vi "Main.vi"(0 "Page Selector":T1, 1 "Code":i32 min=0 max=40000, 4 "Work Area":T2(tab), 5 "Mode Selector":T3, 7 "Instrument Setting":T4={"Error Percentage"=20.0} {"Error Percentage" min=0.0 max=100.0}, 9 "INL Method":T5, 11 "Error In":errorcluster, 12 "Input Voltage Parameters":T6={"Voltage Max"=5.0, "Voltage Min"=0.0, "No.of bits"=3.0} {"No.of bits" min=1.0}) -> (3 "DNL Value":dbl, 6 "DNL Graph":dbl[](graph), 8 "INL Graph":dbl[](graph), 10 "Ideal Transfer Function":cluster{"Analog Voltage":dbl[], dbl[]}(graph), 13 "INL Value":dbl, 14 "Status":string, 15 "Error Out":errorcluster)   [LabVIEW 2023]
doc: "This VI serves as the main entry point for the software framework used to measure INL and DNL for ADC and DAC devices. It initializes the GUI, loads necessary resources, handles user interactions to perform and display measurements."
uses:
  Typedef/INL Method.ctl
  Typedef/Page Selector.ctl
  Typedef/Mode Selector.ctl
  Typedef/Input Voltage Parameters.ctl
  Typedef/Instrument Setting.ctl
  Typedef/Queue Operation.ctl
  Typedef/INL and DNL calculation data.ctl
  Classes/Application/Application.lvclass
  Typedef/Class Details.ctl
  Typedef/Transfer Function.ctl
  Typedef/User Event Operations.ctl
panel:
  in  "Input":bool
  in  "Back":bool
  out "Device Result":string
  # "INL AND DNL TESTS FOR DAC AND ADCs"
  # "Purpose\nThis tool measures Integral Non-Linearity (INL) and Differential Non-Linearity (DNL) of ADCs and DACs, ensuring accurate linearity performance for various applications.\n\nINL and DNL Definitions\nINL (Integral Non-Linearity): Deviation of the converter's actual transfer function from an ideal straight line.\nDNL (Differential Non-Linearity): Deviation between adjacent digital output levels, indicating the uniformity of steps.\n\nA DNL of greater than -1 LSB will guarantee monotonicity and no missing codes.\nMonotonicity\nA device is termed monotonic if the analog output always increases or remains constant as the digital input increases. If the DNL is less than -1 LSB, the transfer function is non-monotonic."
  # "Fig: DNL calculation for ADC"
  # "Please select the mode of the device"
  # "Note: Instrument currently does not work for DAC devices"
  # "Choose the type of INL Measurement"
  # "Specify the error percentage in the limit 0 - 100%"
  # "Please enter the input voltage parameters to generate ideal transfer function"
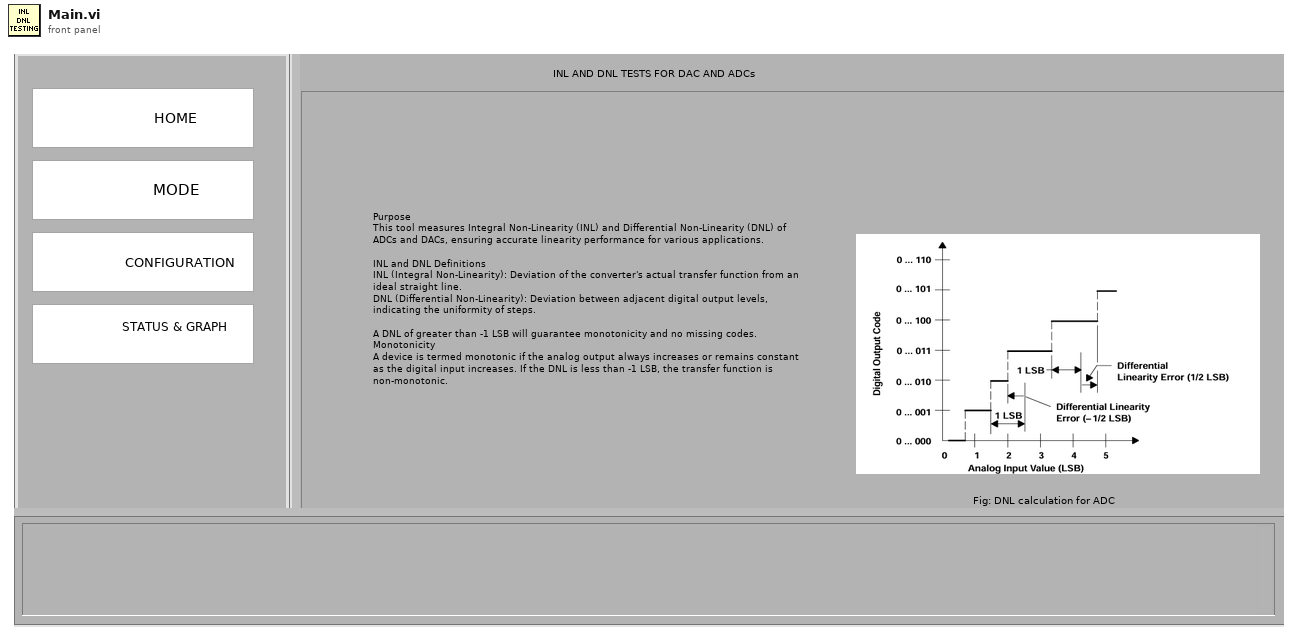
[diagram p1: front panel]
types:
  T1 = typedef "Page Selector.ctl" = cluster{"Mode":bool, "Configuration":bool, "Result":bool, "Home":bool}
  T2 = enum32{"Home Page", "Mode Page", "Configuration Page", "Input Page", "Result Page"}
  T3 = typedef "Mode Selector.ctl" = cluster{"DAC":bool, "ADC":bool}
  T4 = typedef "Instrument Setting.ctl" = cluster{"Error Percentage":dbl}
  T5 = typedef "INL Method.ctl" = enum16{"Best Fit", "End Point"}
  T6 = typedef "Input Voltage Parameters.ctl" = cluster{"Voltage Max":dbl, "Voltage Min":dbl, "No.of bits":dbl}
  T7 = typedef "User Event Operations.ctl" = enum16{"Initialize", "Read", "Write"}
  T8 = typedef "INL and DNL calculation data.ctl" = cluster{"Input Values":T6, "DNL":dbl, "INL":dbl, "DNL Graph":dbl[], "Code":i32, "INL Graph":dbl[], "Error Percentage":dbl, "Status History":string[], "Status Limit":i32, "Statusbar":string, "Active Class":refnum<class "Application.lvclass">, "INL Method":T5, "List of Classes":T9[], "Selected Mode":string, "Base Class":refnum<class "Application.lvclass">, "Transform Function":T10, "Monotonic?":bool, "Device Result":string}
  T9 = typedef "Class Details.ctl" = cluster{"Class Name":string, "Class Data":refnum<class "Application.lvclass">}
  T10 = typedef "Transfer Function.ctl" = cluster{"Ideal voltage":dbl[], "Digital Code":dbl[]}
  T11 = typedef "Queue Operation.ctl" = enum16{"Create & Enqueue N", "Enqueue N", "Dequeue", "Enstack N", "Flush", "Release"}
  T12 = typedef "Queue Element.ctl" = cluster{"State":string, "Data":variant}
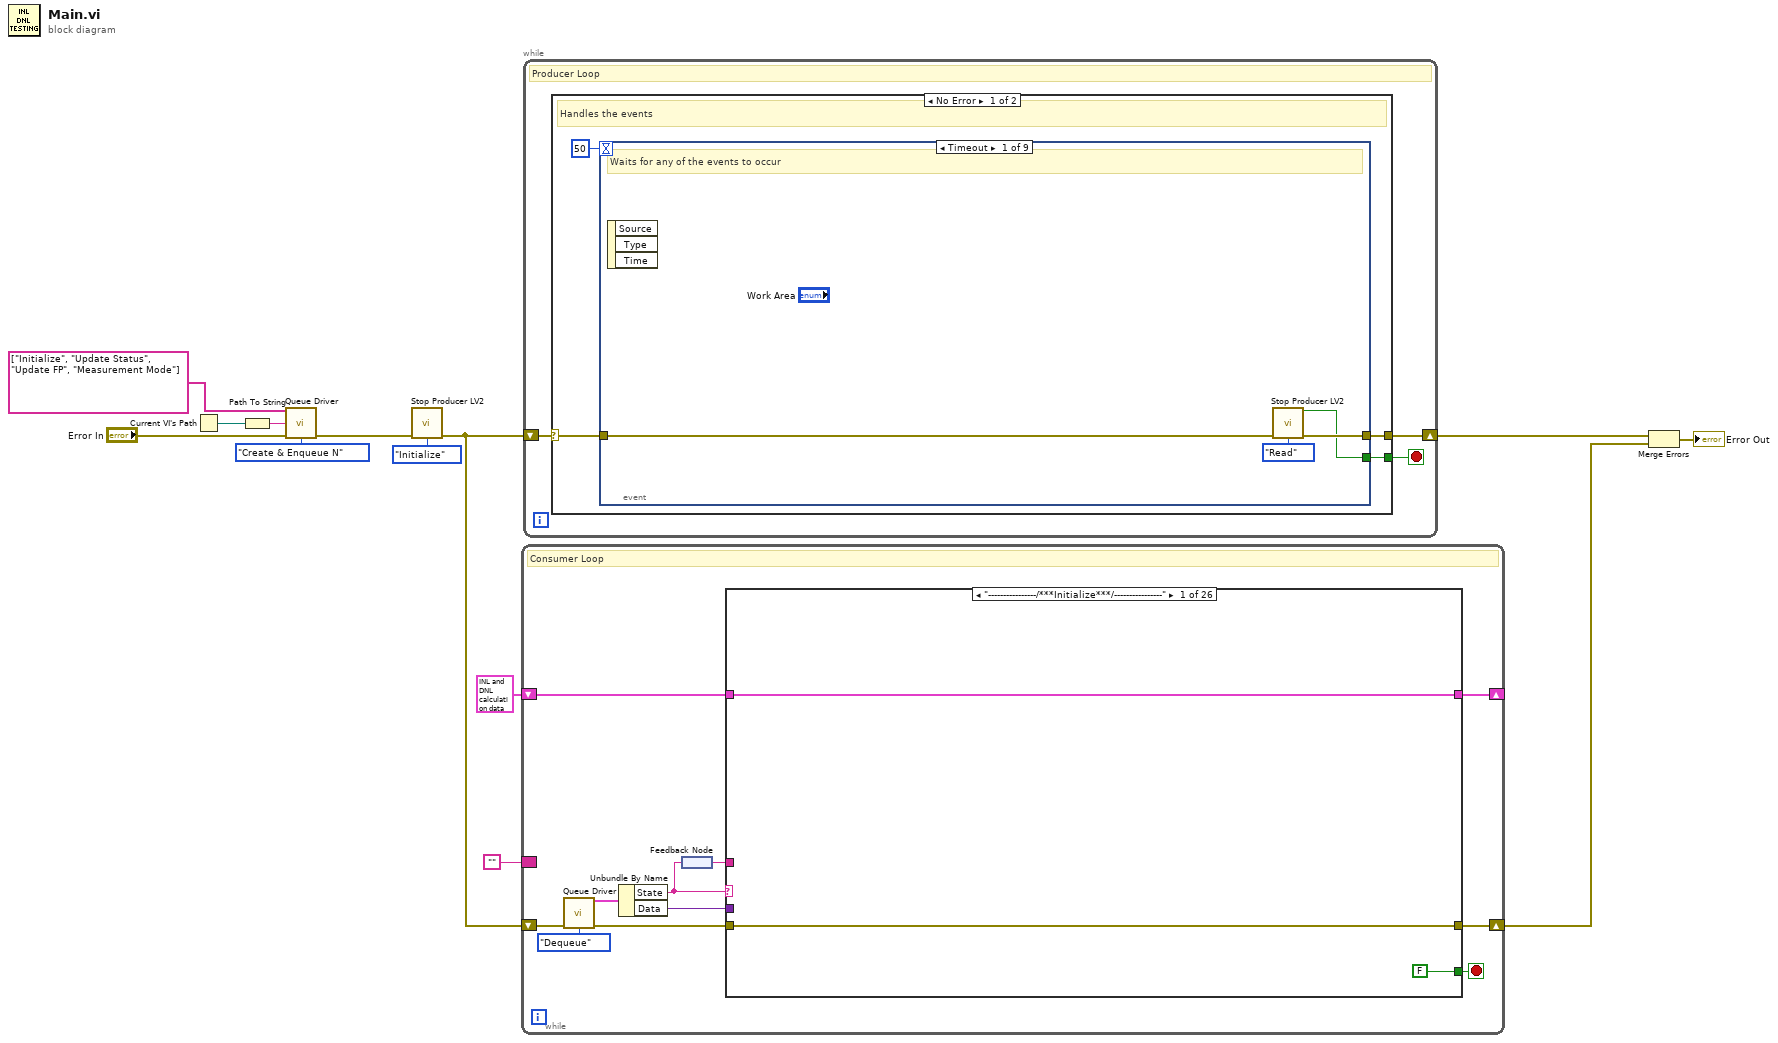
[diagram p0: block diagram]
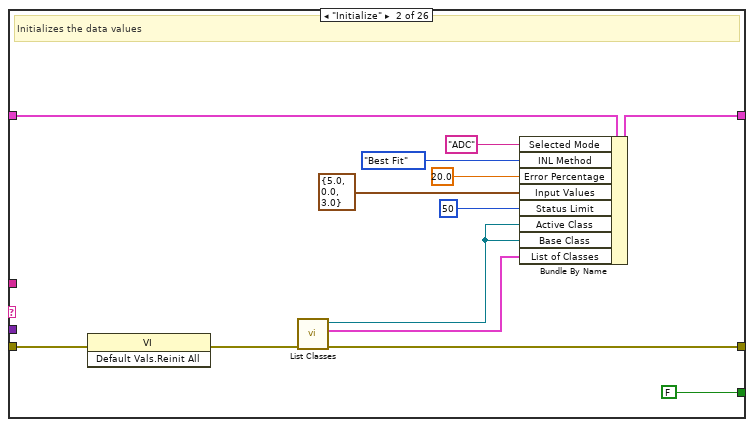
[diagram p2: hidden frame]
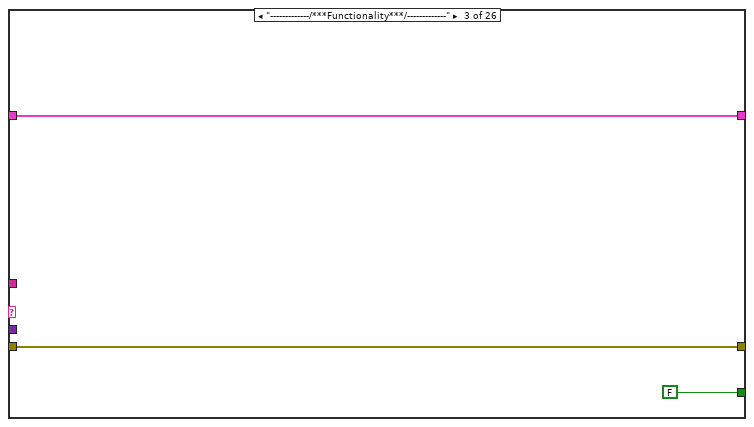
[diagram p3: hidden frame]
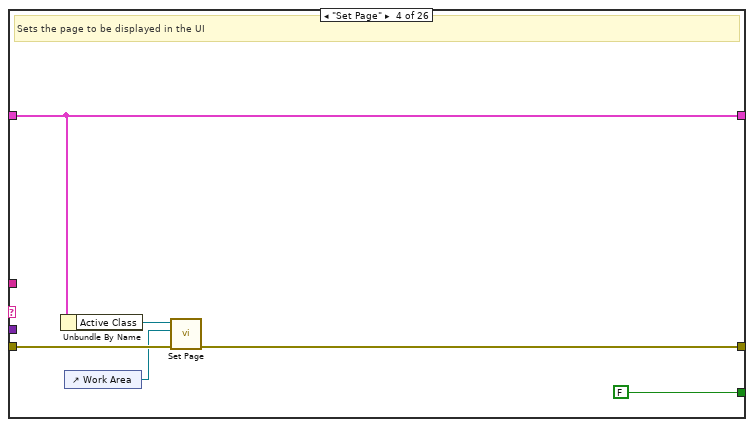
[diagram p4: hidden frame]
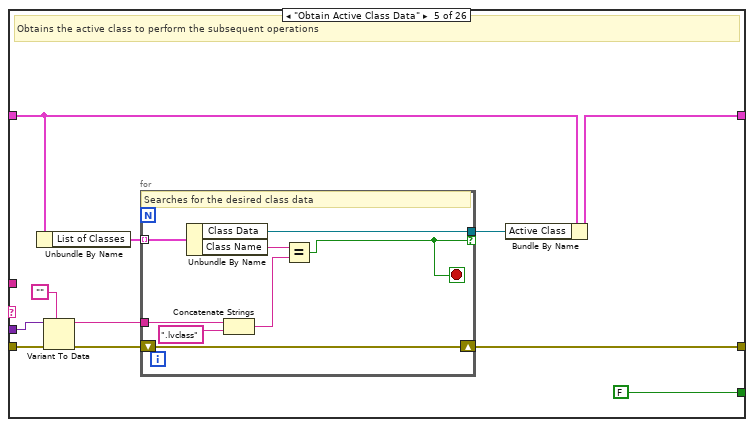
[diagram p5: hidden frame]
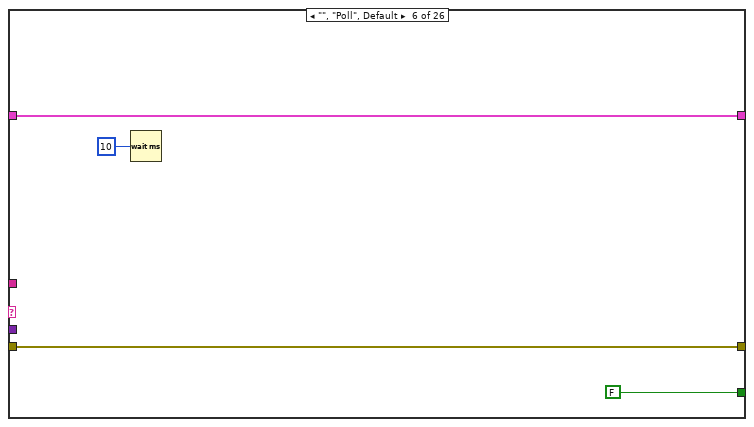
[diagram p6: hidden frame]
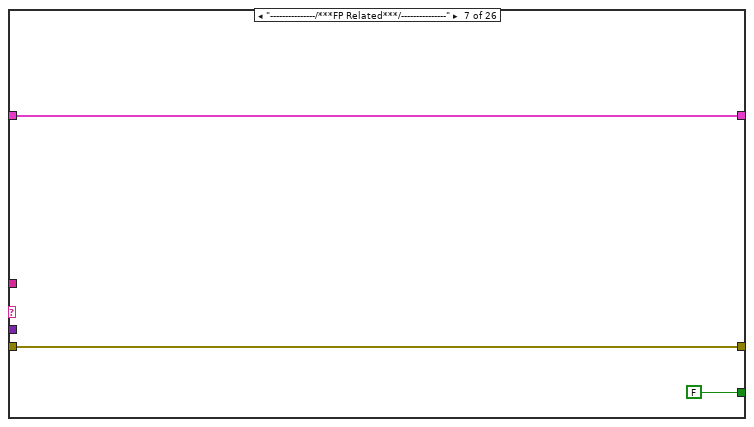
[diagram p7: hidden frame]
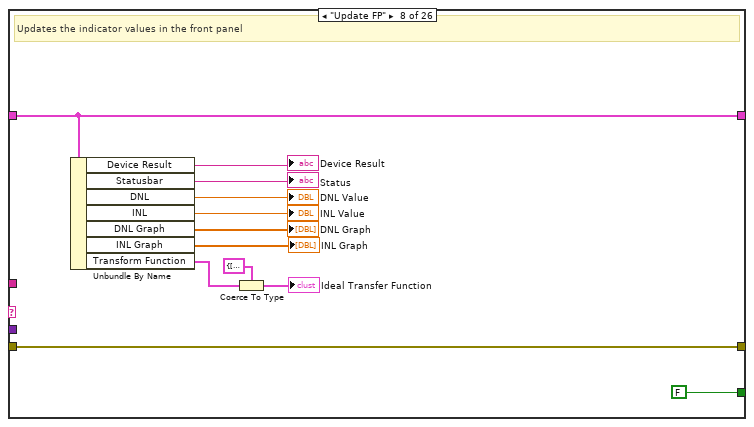
[diagram p8: hidden frame]
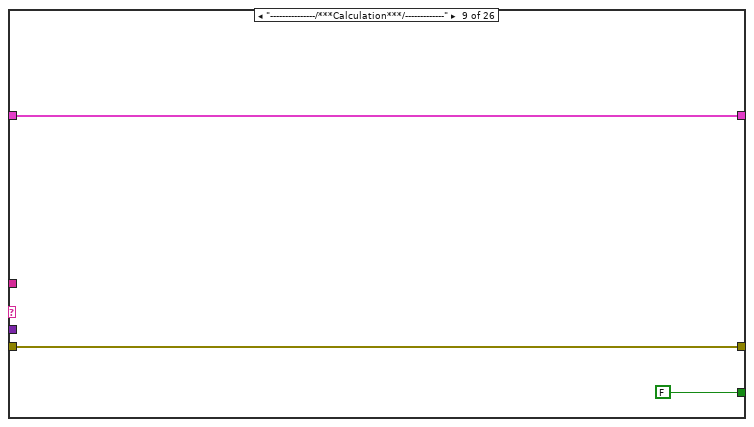
[diagram p9: hidden frame]
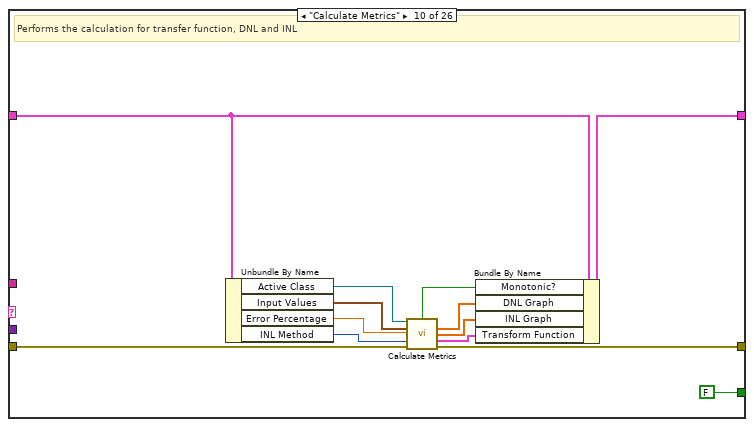
[diagram p10: hidden frame]
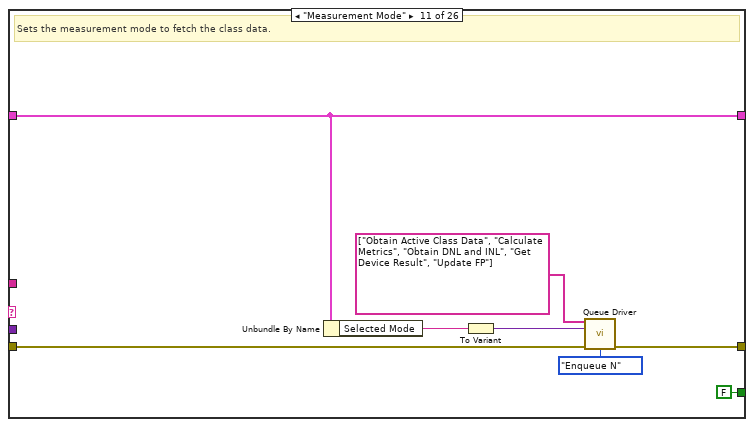
[diagram p11: hidden frame]
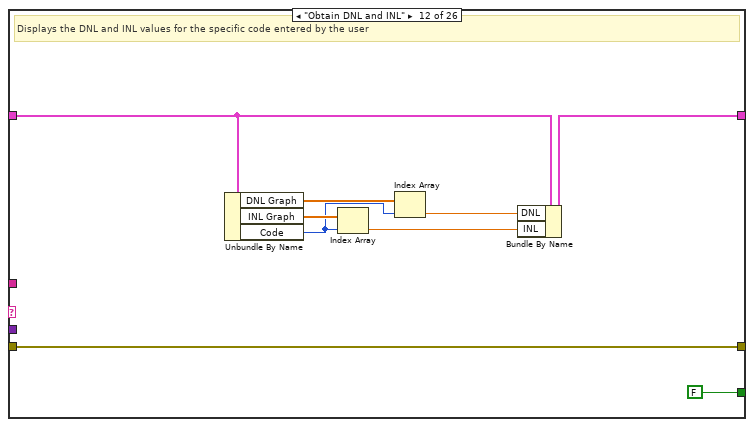
[diagram p12: hidden frame]
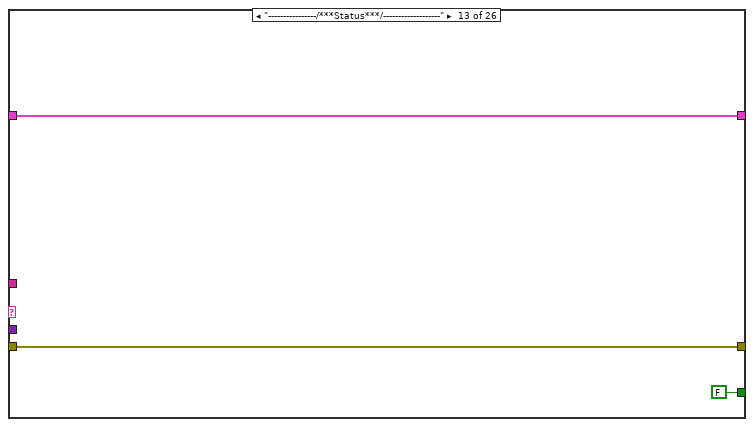
[diagram p13: hidden frame]
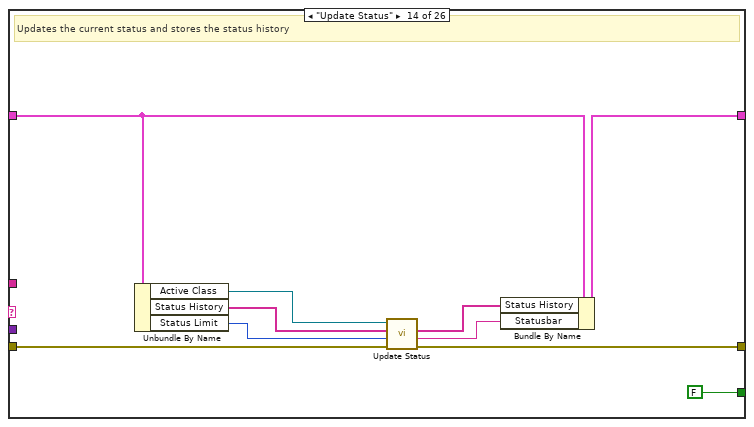
[diagram p14: hidden frame]
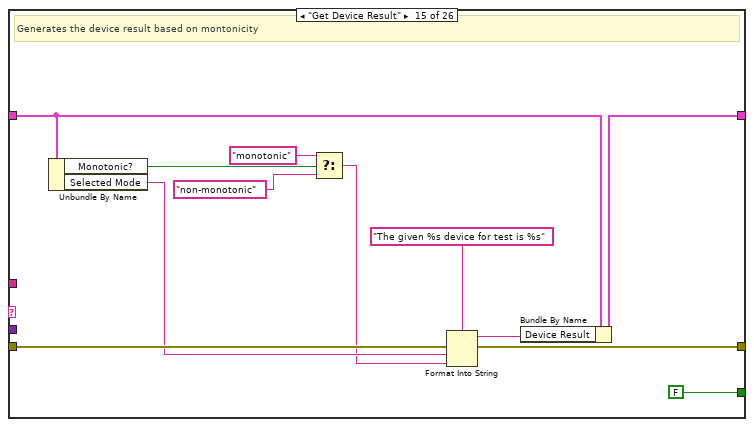
[diagram p15: hidden frame]
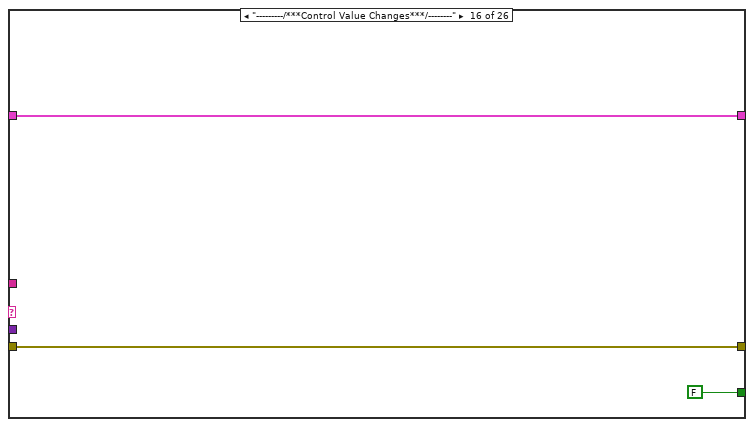
[diagram p16: hidden frame]
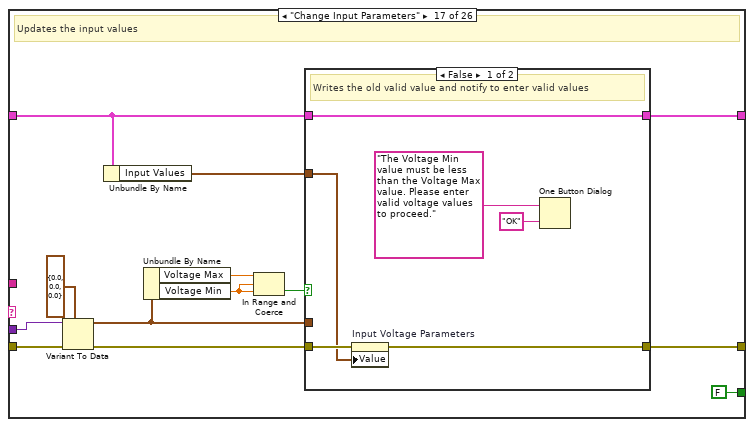
[diagram p17: hidden frame]
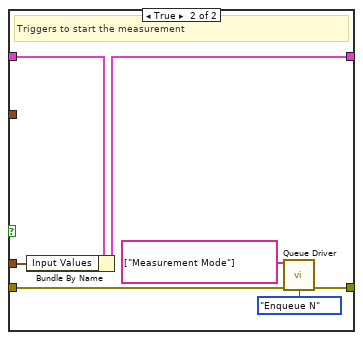
[diagram p18: hidden frame]
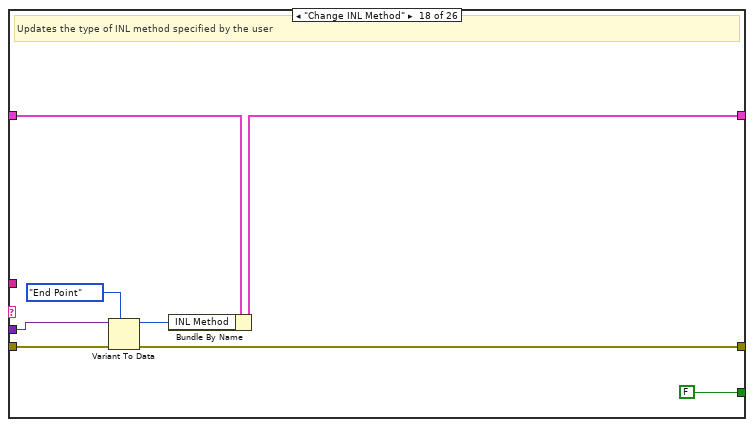
[diagram p19: hidden frame]
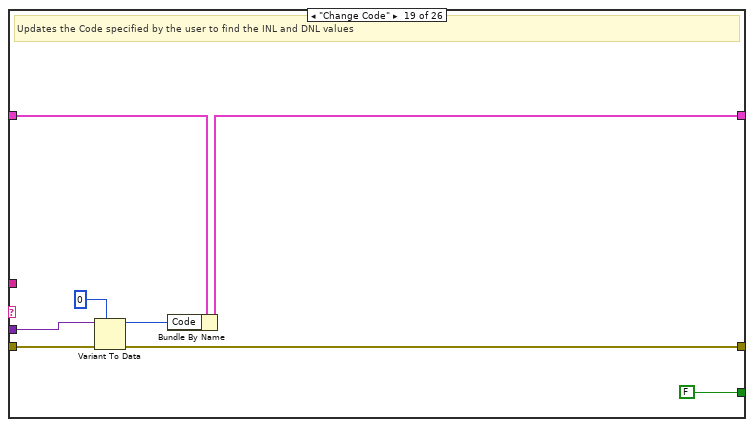
[diagram p20: hidden frame]
diagram:
  n1 = Current VI's Path() -> (path=w5:path)
  n2 = Path To String(path=w5) -> (string=w1:string)
  n3 = call "Queue Driver.vi"("States[]"=string[] ["Initialize", "Update Status", "Update FP", "Measurement Mode"], "Queue Name"=w1, "Error In"="Error In", "Queue Operation"=Queue_Operation."Create & Enqueue N") -> ("Error Out"=w8:errorcluster)  [unwired: 10 in, 1 out]
  n4 = call "Stop Producer LV2.vi"("Error In"=w8, "Operation"=User_Event_Operations."Initialize") -> ("Error Out"=w2:errorcluster)  [unwired: 12 in, 1 out]
  n5 = while {
    shift-right: [w24] -> w13
    shift-left: w2 -> [w21]
    border: "" ("State") -> [_]
    shift-right: [w14] -> _
    shift-left: T8 {"Input Values"={"Voltage Max"=0.0, "Voltage Min"=0.0, "No.of bits"=0.0}, "DNL"=0.0, "INL"=0.0, "DNL Graph"=[], "Code"=0, "INL Graph"=[], "Error Percentage"=0.0, "Status History"=[], "Status Limit"=0, "Statusbar"="", "Active Class"=refnum, "INL Method"=enum."End Point", "List of Classes"=[], "Selected Mode"="", "Base Class"=refnum, "Transform Function"={"Ideal voltage"=[], "Digital Code"=[]}, "Monotonic?"=FALSE, "Device Result"=""} -> [w15]
    stop <- w23 stop-if-true
    # "Consumer Loop"
    n6 = call "Queue Driver.vi"("Error In"=w21, "Queue Operation"=Queue_Operation."Dequeue") -> ("Dequeue Element"=w19:T12, "Error Out"=w20:errorcluster)  [unwired: 12 in]
    n7 = Unbundle By Name(w19) -> ("State"=w17:string, "Data"=w18:variant)
    n8 = feedback-in #1(w17) -> ()
    n9 = feedback #1() -> (w16:string)
    n10 = case shown="\"----------------/***Initialize***/----------------\"" w17 {
      tunnel: [w27 w31 w43 w47 w55 w72 w75 w87 w90 w99 w107 w120 w123 w124 w142 w148 w151 w176 w187 w191 w200 w209 w215 w237 w252 w255] -> w24
      tunnel: [FALSE FALSE FALSE FALSE FALSE FALSE FALSE FALSE FALSE FALSE FALSE FALSE FALSE FALSE FALSE FALSE FALSE FALSE FALSE FALSE FALSE FALSE FALSE FALSE FALSE w253] -> w23
      tunnel: w20 -> [w27 w38 w43 w48 w60 w72 w75 w87 w90 w103 w108 w120 w123 w125 w145 w148 w161 w181 w189 w197 w205 w209 w213 w236 w252 w259]
      tunnel: w18 -> [_ _ _ _ w59 _ _ _ _ _ _ _ _ _ _ _ w159 w179 w186 w195 w203 _ _ w231 _ _]
      tunnel: w16 -> [_ _ _ _ _ _ _ _ _ _ _ _ _ _ _ _ _ _ _ _ _ _ w214 _ _ _]
      tunnel: w15 -> [w26 w39 w42 w46 w53 w71 w74 w85 w89 w102 w105 w117 w122 w132 w144 w147 w150 w182 w190 w198 w206 w208 w210 w235 w251 w256]
      tunnel: [w26 w37 w42 w46 w51 w71 w74 w85 w89 w100 w105 w118 w122 w131 w136 w147 w157 w175 w185 w192 w202 w208 w210 w235 w251 w256] -> w14
      frame "----------------/***Initialize***/----------------" {
      }
      frame "Initialize" {
        # "Initializes the data values"
        n11 = invoke class="VI" method="Default Vals.Reinit All"(error in=w38) -> (error out=w36:errorcluster)  [unwired: 2 in, 2 out]
        n12 = call "List Classes.vi"("Error In"=w36) -> ("Error Out"=w31:errorcluster, "List of classes"=w30:T9[], "Application Out"=w29:refnum<class "Application.lvclass">)  [unwired: 8 in]
        n13 = Bundle By Name(cluster=w39, "Selected Mode"="ADC", "INL Method"=INL_Method."Best Fit", "Error Percentage"=20.0, "Input Values"=T6 {"Voltage Max"=5.0, "Voltage Min"=0.0, "No.of bits"=3.0}, "Status Limit"=50, "Active Class"=w29, "Base Class"=w29, "List of Classes"=w30) -> (w37:T8)
      }
      frame "-------------/***Functionality***/-------------" {
      }
      frame "Set Page" {
        # "Sets the page to be displayed in the UI"
        n14 = Unbundle By Name(w46) -> ("Active Class"=w44:refnum<class "Application.lvclass">)
        n15 = control-ref of="Work Area"() -> (w45:refnum<vi>)
        n16 = call "Set Page.vi"("Error In"=w48, "Tab Control"=w45, "Application In"=w44) -> ("Error Out"=w47:errorcluster)  [unwired: 7 in, 1 out]
      }
      frame "Obtain Active Class Data" {
        # "Obtains the active class to perform the subsequent operations"
        n17 = Unbundle By Name(w53) -> ("List of Classes"=w52:T9[])
        n18 = Variant To Data(error in=w60, type="", Variant=w59) -> (data=w54:string, error out=w56:errorcluster)
        n19 = for {
          shift-right: [w68] -> w55
          shift-left: w56 -> [w68]
          tunnel: w54 -> [w65]
          tunnel: w52 -> [w67] mode=indexing
          tunnel: [w64] -> w50 if=w63
          stop <- w63 stop-if-true
          # "Searches for the desired class data"
          n20 = Unbundle By Name(w67) -> ("Class Data"=w64:refnum<class "Application.lvclass">, "Class Name"=w66:string)
          n21 = Concatenate Strings(w65, ".lvclass" ("string")) -> (w62:string)
          n22 = Equal?(x=w66, y=w62) -> (x = y?=w63:bool)
        }
        n23 = Bundle By Name(cluster=w53, "Active Class"=w50) -> (w51:T8)
      }
      frame "", "Poll", Default {
        n24 = Wait (ms)(milliseconds to wait=u32 10 ("millisecond timer value")) -> ()  [unwired: 1 out]
      }
      frame "---------------/***FP Related***/---------------" {
      }
      frame "Update FP" {
        # "Updates the indicator values in the front panel"
        n25 = Unbundle By Name(w85) -> ("Device Result"=→"Device Result":string, "Statusbar"=→"Status":string, "DNL"=→"DNL Value":dbl, "INL"=→"INL Value":dbl, "DNL Graph"=→"DNL Graph":dbl[], "INL Graph"=→"INL Graph":dbl[], "Transform Function"=w84:T10)
        n26 = Coerce To Type(0:w84, 1:cluster{"Analog Voltage":dbl[], dbl[]} {"Analog Voltage"=[0.625, 1.25, 1.875, 2.5, 3.125, 3.75, 4.375, 5.0], [1.0, 2.0, 3.0, 4.0, 5.0, 6.0, 7.0, 8.0]} ("Ideal Transfer Function")) -> (2:→"Ideal Transfer Function":cluster{"Analog Voltage":dbl[], dbl[]})
      }
      frame "---------------/***Calculation***/-------------" {
      }
      frame "Calculate Metrics" {
        # "Performs the calculation for transfer function, DNL and INL"
        n27 = Unbundle By Name(w102) -> ("Active Class"=w97:refnum<class "Application.lvclass">, "Input Values"=w98:T6, "Error Percentage"=w95:dbl, "INL Method"=w96:T5)
        n28 = call "Calculate Metrics.vi"("Application In"=w97, "Input Values"=w98, "Error Percentage"=w95, "INL Method"=w96, "Error In"=w103) -> ("Monotonic?"=w91:bool, "DNL Values"=w94:dbl[], "INL Values"=w93:dbl[], "Transfer Function"=w92:T10, "Error Out"=w99:errorcluster)  [unwired: 5 in, 1 out]
        n29 = Bundle By Name(cluster=w102, "Monotonic?"=w91, "DNL Graph"=w94, "INL Graph"=w93, "Transform Function"=w92) -> (w100:T8)
      }
      frame "Measurement Mode" {
        # "Sets the measurement mode to fetch the class data."
        n30 = Unbundle By Name(w105) -> ("Selected Mode"=w109:string)
        n31 = To Variant(anything=w109) -> (Variant=w104:variant)
        n32 = call "Queue Driver.vi"("States[]"=string[] ["Obtain Active Class Data", "Calculate Metrics", "Obtain DNL and INL", "Get Device Result", "Update FP"], "Data"=w104, "Error In"=w108, "Queue Operation"=Queue_Operation."Enqueue N") -> ("Error Out"=w107:errorcluster)  [unwired: 10 in, 1 out]
      }
      frame "Obtain DNL and INL" {
        # "Displays the DNL and INL values for the specific code entered by the user"
        n33 = Unbundle By Name(w117) -> ("DNL Graph"=w115:dbl[], "INL Graph"=w116:dbl[], "Code"=w114:i32)
        n34 = Index Array(array=w116, index=w114) -> (element=w112:dbl)
        n35 = Index Array(array=w115, index=w114) -> (element=w113:dbl)
        n36 = Bundle By Name(cluster=w117, "DNL"=w113, "INL"=w112) -> (w118:T8)
      }
      frame "----------------/***Status***/-------------------" {
      }
      frame "Update Status" {
        # "Updates the current status and stores the status history"
        n37 = Unbundle By Name(w132) -> ("Active Class"=w128:refnum<class "Application.lvclass">, "Status History"=w129:string[], "Status Limit"=w130:i32)
        n38 = call "Update Status.vi"("Error In"=w125, "Status Limit"=w130, "Status History In"=w129, "Application In"=w128) -> ("Error Out"=w124:errorcluster, "Status"=w126:string, "Status History Out"=w127:string[])  [unwired: 2 in, 1 out]
        n39 = Bundle By Name(cluster=w132, "Status History"=w127, "Statusbar"=w126) -> (w131:T8)
      }
      frame "Get Device Result" {
        # "Generates the device result based on montonicity"
        n40 = Unbundle By Name(w144) -> ("Monotonic?"=w143:bool, "Selected Mode"=w141:string)
        n41 = Select(t="monotonic", s=w143, f="non-monotonic") -> (s? t:f=w139:string)
        n42 = Format Into String(format string="The given %s device for test is %s", error in=w145, w141, w139) -> (resulting string=w135:string, error out=w142:errorcluster)  [unwired: 1 in]
        n43 = Bundle By Name(cluster=w144, "Device Result"=w135) -> (w136:T8)
      }
      frame "---------/***Control Value Changes***/--------" {
      }
      frame "Change Input Parameters" {
        # "Updates the input values"
        n44 = Variant To Data(error in=w161, type=T6 {"Voltage Max"=0.0, "Voltage Min"=0.0, "No.of bits"=0.0} ("Input Values"), Variant=w159) -> (data=w156:T6, error out=w152:errorcluster)
        n45 = Unbundle By Name(w150) -> ("Input Values"=w149:T6)
        n46 = Unbundle By Name(w156) -> ("Voltage Max"=w155:dbl, "Voltage Min"=w154:dbl)
        n47 = In Range and Coerce(upper limit=w155, x=w154, lower limit=w154) -> (In Range?=w153:bool)  [unwired: 1 out]
        n48 = case shown="False" w153 {
          tunnel: w150 -> [w167 w174]
          tunnel: [w167 w173] -> w157
          tunnel: w156 -> [_ w172]
          tunnel: w152 -> [w165 w171]
          tunnel: [w163 w170] -> w151
          tunnel: w149 -> [w162 _]
          frame False {
            # "Writes the old valid value and notify to enter valid values"
            n49 = property on="Input Voltage Parameters" class="Clust (strict)"(error in=w165, "Value"=w162) -> (error out=w163:errorcluster)  [unwired: 1 in, 1 out]
            n50 = One Button Dialog(message="The Voltage Min value must be less than the Voltage Max value. Please enter valid voltage values to proceed.", button name ("OK")="OK") -> ()  [unwired: 1 out]
          }
          frame True {
            # "Triggers to start the measurement"
            n51 = Bundle By Name(cluster=w174, "Input Values"=w172) -> (w173:T8)
            n52 = call "Queue Driver.vi"("States[]"=string[] ["Measurement Mode"], "Error In"=w171, "Queue Operation"=Queue_Operation."Enqueue N") -> ("Error Out"=w170:errorcluster)  [unwired: 11 in, 1 out]
          }
        }
      }
      frame "Change INL Method" {
        # "Updates the type of INL method specified by the user"
        n53 = Variant To Data(error in=w181, type=INL_Method."End Point" ("NewVal"), Variant=w179) -> (data=w177:T5, error out=w176:errorcluster)
        n54 = Bundle By Name(cluster=w182, "INL Method"=w177) -> (w175:T8)
      }
      frame "Change Code" {
        # "Updates the Code specified by the user to find the INL and DNL values"
        n55 = Variant To Data(error in=w189, type=0 ("Code"), Variant=w186) -> (data=w184:i32, error out=w187:errorcluster)
        n56 = Bundle By Name(cluster=w190, "Code"=w184) -> (w185:T8)
      }
      frame "Change Error" {
        # "Updates the error percentage specified by the user"
        n57 = Variant To Data(error in=w197, type=0.0 ("Code"), Variant=w195) -> (data=w194:dbl, error out=w191:errorcluster)
        n58 = Bundle By Name(cluster=w198, "Error Percentage"=w194) -> (w192:T8)
      }
      frame "Change Mode" {
        # "Updates the changed mode value"
        n59 = Variant To Data(error in=w205, type="", Variant=w203) -> (data=w199:string, error out=w200:errorcluster)
        n60 = Bundle By Name(cluster=w206, "Selected Mode"=w199) -> (w202:T8)
      }
      frame "------------------/***Error***/-----------------" {
      }
      frame "Error" {
        # "Handles the error based on the user acknowledgement"
        n61 = Unbundle By Name(w213) -> ("code"=w212:i32, "source"=w211:string)
        n62 = call <vilib>:"Clear Errors.vi"("error in (no error)"=w213) -> ("error out"=w222:errorcluster)  [unwired: 5 in, 1 out]
        n63 = Format Into String(format string="Error occurred in state \"%s\"!!\nError Code: %d\nError Source: %s\n\nDo you wish to continue?", error in=w222, w214, w212, w211) -> (resulting string=w220:string, error out=w216:errorcluster)  [unwired: 1 in]
        n64 = Two Button Dialog(message=w220, 1:"Exit" ("F button name (\"Cancel\")"), 2:"Continue" ("T button name (\"OK\")")) -> (T button?=w217:bool)
        n65 = case "Continue?" shown="False" w217 {
          tunnel: w216 -> [w227 w228]
          tunnel: [w226 w228] -> w215
          frame False {
            # "Enqueues exit state to stop the VI running"
            n66 = call "Queue Driver.vi"("States[]"=string[] ["Exit"], "Error In"=w227, "Queue Operation"=Queue_Operation."Enstack N") -> ("Error Out"=w226:errorcluster)  [unwired: 11 in, 1 out]
          }
          frame True {
            # "Continues the process"
          }
        }
      }
      frame "Producer Error" {
        # "Handles the producer error based on the user acknowledgement"
        n67 = Variant To Data(error in=w236, type=errorcluster {"status"=FALSE, "code"=0, "source"=""} ("error out"), Variant=w231) -> (data=w229:errorcluster, error out=w232:errorcluster)
        n68 = Unbundle By Name(w229) -> ("code"=w234:i32, "source"=w233:string)
        n69 = Format Into String(format string="Error occurred!\nError Code: %d\nError Source: %s\n\nDo you wish to continue?", error in=w232, w234, w233) -> (resulting string=w242:string, error out=w238:errorcluster)  [unwired: 1 in]
        n70 = Two Button Dialog(message=w242, 1:"Exit" ("F button name (\"Cancel\")"), 2:"Continue" ("T button name (\"OK\")")) -> (T button?=w239:bool)
        n71 = case "Continue?" shown="False" w239 {
          tunnel: w238 -> [w248 w249]
          tunnel: [w247 w249] -> w237
          frame False {
            # "Enqueues exit state to stop the VI running"
            n72 = call "Queue Driver.vi"("States[]"=string[] ["Exit"], "Error In"=w248, "Queue Operation"=Queue_Operation."Enstack N") -> ("Error Out"=w247:errorcluster)  [unwired: 11 in, 1 out]
          }
          frame True {
            # "Continues the process"
          }
        }
      }
      frame "-----------------/***Exit***/------------------" {
      }
      frame "Exit" {
        w253 = TRUE
        # "Releases the queue and stops the consumer loop running"
        n73 = call "Queue Driver.vi"("Error In"=w259, "Queue Operation"=Queue_Operation."Flush") -> ("Error Out"=w258:errorcluster)  [unwired: 12 in, 1 out]
        n74 = call "Queue Driver.vi"("Error In"=w258, "Queue Operation"=Queue_Operation."Release") -> ("Error Out"=w257:errorcluster)  [unwired: 12 in, 1 out]
        n75 = call "Stop Producer LV2.vi"("Stop"=w253, "Error In"=w257, "Operation"=User_Event_Operations."Write") -> ("Error Out"=w255:errorcluster)  [unwired: 11 in, 1 out]
      }
    }
  }
  n76 = while {
    shift-right: [w262] -> w10
    shift-left: w2 -> [w264]
    stop <- w263 stop-if-true
    # "Producer Loop"
    n77 = case shown="No Error" w264 {
      selector: w264 -> [w268 w339]
      tunnel: [w267 FALSE ("Stop")] -> w263
      tunnel: [w265 w337] -> w262
      frame No Error {
        # "Handles the events"
        n78 = event shown="[0] Timeout" {
          selector: _ -> [_ _ _ _ _ _ _ _ _]
          dyn-events: _ -> [_ _ _ _ _ _ _ _ _]
          timeout: 50 -> [_ _ _ _ _ _ _ _ _]
          tunnel: w268 -> [w272 w286 w290 w297 w302 w310 w320 w324 w332]
          tunnel: [w269 FALSE ("Stop") FALSE ("Stop") FALSE ("Stop") FALSE ("Stop") FALSE ("Stop") FALSE ("Stop") FALSE ("Stop") w328] -> w267
          tunnel: [w271 w282 w289 w296 w301 w311 w317 w322 w331] -> w265
          event Timeout {
            # "Waits for any of the events to occur"
            n79 = event-data() -> ()  [unwired: 1 in, 3 out]
            n80 = call "Stop Producer LV2.vi"("Error In"=w272, "Operation"=User_Event_Operations."Read") -> ("Stop"=w269:bool, "Error Out"=w271:errorcluster)  [unwired: 12 in]
          }
          event "Input": Value Change {
            w276 = TRUE ("Key Focus")
            # "Obtains the name of the control clicked and navigates to the respective page"
            n81 = event-data() -> ("CtlRef"=w279:refnum<vi>)  [unwired: 1 in]
            n82 = property on="Page Selector" class="Clust (strict)"(error in=w286, "Value"=T1 {"Mode"=FALSE, "Configuration"=FALSE, "Result"=FALSE, "Home"=FALSE} ("Page Selector")) -> (error out=w278:errorcluster)  [unwired: 1 in, 1 out]
            n83 = property on="Input" class="Bool (strict)"(error in=w278, "Value"=FALSE ("Input")) -> (error out=w274:errorcluster)  [unwired: 1 in, 1 out]
            n84 = property class="Bool (strict)"(reference=w279, error in=w274, "Key Focus"=w276, "Value"=w276) -> (error out=w283:errorcluster, "Label.Text"=w275:string)  [unwired: 1 out]
            n85 = To Variant(anything=w275) -> (Variant=w280:variant)
            n86 = call "Queue Driver.vi"("States[]"=string[] ["Obtain Active Class Data", "Set Page", "Update Status", "Update FP"], "Data"=w280, "Error In"=w283, "Queue Operation"=Queue_Operation."Enqueue N") -> ("Error Out"=w282:errorcluster)  [unwired: 10 in, 1 out]
          }
          event Value Change {
            # "Updates the input voltage paramaters values"
            n87 = event-data() -> ("NewVal"=w292:T6)  [unwired: 1 in]
            n88 = To Variant(anything=w292) -> (Variant=w287:variant)
            n89 = call "Queue Driver.vi"("States[]"=string[] ["Change Input Parameters"], "Data"=w287, "Error In"=w290, "Queue Operation"=Queue_Operation."Enqueue N") -> ("Error Out"=w289:errorcluster)  [unwired: 10 in, 1 out]
          }
          event "Back": Value Change {
            # "Navigates back to the mode selection page"
            n90 = event-data() -> ()  [unwired: 1 in, 1 out]
            n91 = property on="Mode" class="Bool (strict)"(error in=w297, "Val(Sgnl)"=TRUE ("Value (Signaling)")) -> (error out=w296:errorcluster)  [unwired: 1 in, 1 out]
          }
          event Value Change {
            # "Updates the type of INL measurement method selected by the user"
            n92 = event-data() -> ("NewVal"=w300:T5)  [unwired: 1 in]
            n93 = To Variant(anything=w300) -> (Variant=w298:variant)
            n94 = call "Queue Driver.vi"("States[]"=string[] ["Change INL Method", "Measurement Mode"], "Data"=w298, "Error In"=w302, "Queue Operation"=Queue_Operation."Enqueue N") -> ("Error Out"=w301:errorcluster)  [unwired: 10 in, 1 out]
          }
          event Value Change {
            # "Obtains the mode selected by the user and triggers to navigate  to the input page."
            n95 = event-data() -> ("CtlRef"=w308:refnum<vi>)  [unwired: 1 in]
            n96 = property class="Bool (strict)"(reference=w308, error in=w310) -> (error out=w309:errorcluster, "Label.Text"=w307:string)  [unwired: 1 out]
            n97 = To Variant(anything=w307) -> (Variant=w305:variant)
            n98 = call "Queue Driver.vi"("States[]"=string[] ["Change Mode", "Measurement Mode"], "Data"=w305, "Error In"=w309, "Queue Operation"=Queue_Operation."Enqueue N") -> ("Error Out"=w311:errorcluster)  [unwired: 10 in, 1 out]
          }
          event "Code": Value Change {
            # "Updates the new code value to display the INL and DNL values respectively"
            n99 = event-data() -> ("NewVal"=w316:i32)  [unwired: 1 in]
            n100 = To Variant(anything=w316) -> (Variant=w314:variant)
            n101 = call "Queue Driver.vi"("States[]"=string[] ["Change Code", "Obtain DNL and INL", "Update FP"], "Data"=w314, "Error In"=w320, "Queue Operation"=Queue_Operation."Enqueue N") -> ("Error Out"=w317:errorcluster)  [unwired: 10 in, 1 out]
          }
          event Value Change {
            # "Updates the change in error value"
            n102 = event-data() -> ("NewVal"=w325:dbl)  [unwired: 1 in]
            n103 = To Variant(anything=w325) -> (Variant=w321:variant)
            n104 = call "Queue Driver.vi"("States[]"=string[] ["Change Error", "Measurement Mode"], "Data"=w321, "Error In"=w324, "Queue Operation"=Queue_Operation."Enqueue N") -> ("Error Out"=w322:errorcluster)  [unwired: 10 in, 1 out]
          }
          event Panel Close? {
            w329 = TRUE ("Discard?")
            # "Stops the VI running when user clicks panel close"
            n105 = event-data() -> ()  [unwired: 1 in, 1 out]
            n106 = call "Queue Driver.vi"("States[]"=string[] ["Exit"], "Error In"=w332, "Queue Operation"=Queue_Operation."Enstack N") -> ("Error Out"=w331:errorcluster)  [unwired: 11 in, 1 out]
            n107 = event-data("Discard?"=w329) -> ()  [unwired: 1 in, 1 out]
            n108 = Not(x=w329) -> (.not. x?=w328:bool)
          }
        }
      }
      frame Error {
        # "Passes the error to the consumer loop"
        n109 = Unbundle By Name(w339) -> ("code"=w340:i32)
        n110 = To Variant(anything=w339) -> (Variant=w334:variant)
        n111 = call <vilib>:"Clear Errors.vi"("error in (no error)"=w339, "specific error code to clear (0: all)"=w340) -> ("error out"=w338:errorcluster)  [unwired: 4 in, 1 out]
        n112 = call "Queue Driver.vi"("States[]"=string[] ["Producer Error"], "Data"=w334, "Error In"=w338, "Queue Operation"=Queue_Operation."Enqueue N") -> ("Error Out"=w337:errorcluster)  [unwired: 10 in, 1 out]
      }
    }
  }
  n113 = Merge Errors(w10, w13) -> (→"Error Out":errorcluster)
